vi "GetPropertyObject.vi"(8 "error in (no error)":errorcluster, 10 "lookup string":string, 11 "property object in":refnum<k7>) -> (0 "error out":errorcluster, 1 "exists":bool, 2 "property object":refnum<k7>, 3 "property object out":refnum<k7>)   [LabVIEW 2019]
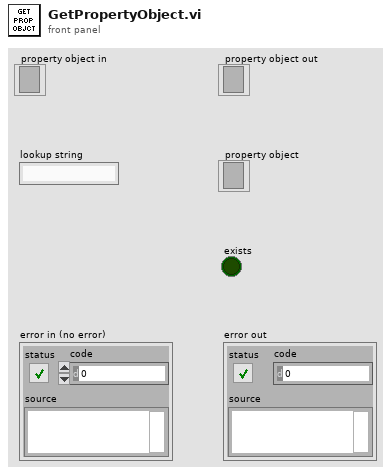
[diagram p1: front panel]
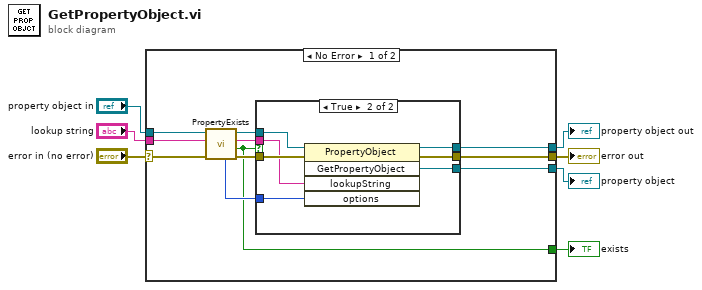
[diagram p0: block diagram]
diagram:
  n1 = case shown="No Error" "error in (no error)" {
    selector: "error in (no error)" -> [w12 w28]
    tunnel: [w18 w29] -> w7
    tunnel: [w17 w28] -> w6
    tunnel: "lookup string" -> [w15 _]
    tunnel: "property object in" -> [w13 w29]
    tunnel: [w11 _] -> w2
    tunnel: [w8 _] -> w1
    frame No Error {
      n2 = call "PropertyExists.vi"("error in (no error)"=w12, "lookup string in"=w15, "property object in"=w13) -> ("error out"=w16:errorcluster, "exists"=w8:bool, "lookup string out"=w10:string, "property object out"=w14:refnum<k7>, "options"=w9:i32)  [unwired: 4 in]
      n3 = case shown="True" w8 {
        tunnel: w14 -> [w19 w26]
        tunnel: w10 -> [_ w25]
        tunnel: w16 -> [w20 w27]
        tunnel: [_ w24] -> w11
        tunnel: [w20 w23] -> w17
        tunnel: [w19 w22] -> w18
        tunnel: w9 -> [_ w21]
        frame False {
        }
        frame True {
          n4 = invoke class="PropertyObject" method="GetPropertyObject"(reference=w26, error in=w27, "lookupString"=w25, "options"=w21) -> (reference out=w22:refnum<k7>, error out=w23:errorcluster, "GetPropertyObject"=w24:refnum<k7>)  [unwired: 1 in, 2 out]
        }
      }
    }
    frame Error {
    }
  }
  "property object out" <- w7
  "error out" <- w6
  "property object" <- w2
  "exists" <- w1
